vi "List_Inst_Positions.vi"() -> (0 "Position Info":string[][](array[string]))   [LabVIEW 2011]
uses:
  Anemometry/Anemometry Sub Vis/Globals/Meas_global.vi
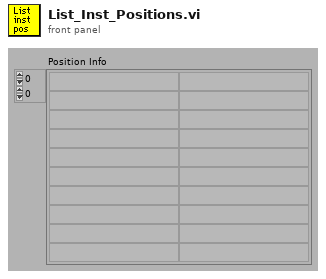
[diagram p1: front panel]
types:
  T1 = typedef "Analysis_info_cluster.ctl" = cluster{"Colour":u32, "Inst type":T2, "Inst name":string, "Symbol":string, "Code name":string, "Extra Info":string, "Inst Array":T3, "Index":i32, "Voltage Index":i32, "Extra Titles":string[], "Extra Values":string[], "Eng Values":dbl[], "Time (ms)":dbl[], "Voltage":dbl[], "U":dbl, "u^2":dbl, "u^3":dbl, "u^4":dbl, "Skew_u":dbl, "Kurt_u":dbl, "Sd Error in Mean":dbl, "% u'/U":dbl, "X":dbl, "Y":dbl, "Z":dbl, "Spectra":T4, "Autocorrelation":T4, "Timescale integral to 25%":dbl, "Sd Error in Variance":dbl, "Calib File":path, "Calib Constants":dbl[], "Histogram":T4, "Output Position":bool, "Full Stats":bool, "Weighting":dbl[]}
  T2 = typedef "Inst_type.ctl" = enum16{"Propeller anemometer", "Raw voltage", "Pressure Transducer", "Pitot-static tube", "Preston tube", "Hot wire", "Cross wire 1", "Cross wire 2", "Generic Linear", "Generic Polynomial", "Generic BackPoly", "Fast FID", "Thermocouple", "Cold wire", "Pulsed Wire", "LDA Vel", "LDA Tran time", "LDA Arr time"}
  T3 = typedef "Instrument_Array.ctl" = enum16{"PWA", "LDA", "Analogue"}
  T4 = typedef "XY_Plot_Cluster.ctl" = cluster{"First Name":string, "Second Name":string, "X axis name":string, "Y axis name":string, "X array":dbl[], "Y array":dbl[]}
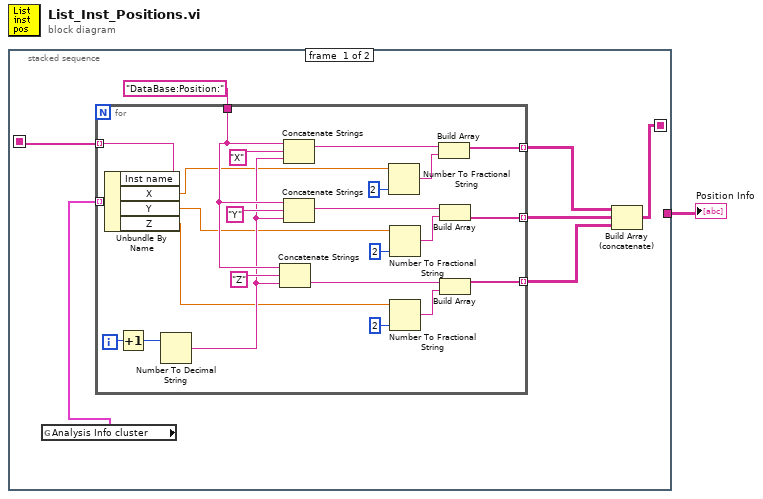
[diagram p0: block diagram]
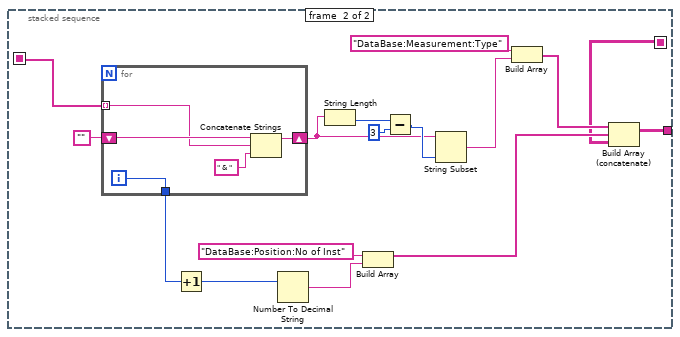
[diagram p2: hidden frame]
diagram:
  n1 = stacked-sequence {
    seq-local: [w4 _] -> [_ w34]
    seq-local: [w3 _] -> [_ w44]
    tunnel: [_ w33] -> w1
    frame #0 {
      n2 = global read "Meas_global.vi" "Analysis Info cluster"() -> (w2:T1[])
      n3 = for {
        tunnel: w2 -> [w32] mode=indexing
        tunnel: "DataBase:Position:" -> [w29]
        tunnel: [w13] -> w7 mode=indexing
        tunnel: [w12] -> w6 mode=indexing
        tunnel: [w11] -> w5 mode=indexing
        tunnel: [w9] -> w3 mode=indexing
        i -> [w30]
        n4 = Unbundle By Name(w32) -> ("Inst name"=w9:string, "X"=w22:dbl, "Y"=w16:dbl, "Z"=w15:dbl)
        n5 = Increment(x=w30) -> (x+1=w10:i32)
        n6 = Number To Decimal String(number=w10) -> (decimal integer string=w26:string)  [unwired: 1 out]
        n7 = Concatenate Strings(w29, "Z", w26) -> (w14:string)
        n8 = Concatenate Strings(w29, "X", w26) -> (w25:string)
        n9 = Concatenate Strings(w29, "Y", w26) -> (w17:string)
        n10 = Number To Fractional String(number=w22, precision (6)=i16 2) -> (F-format string=w23:string)  [unwired: 2 out]
        n11 = Number To Fractional String(number=w16, precision (6)=i16 2) -> (F-format string=w21:string)  [unwired: 2 out]
        n12 = Number To Fractional String(number=w15, precision (6)=i16 2) -> (F-format string=w18:string)  [unwired: 2 out]
        n13 = Build Array(w25, w23) -> (w12:string[])
        n14 = Build Array(w17, w21) -> (w13:string[])
        n15 = Build Array(w14, w18) -> (w11:string[])
      }
      n16 = Build Array (concatenate)(w6, w7, w5) -> (w4:string[][])
    }
    frame #1 {
      n17 = for {
        shift-right: [w52] -> w40
        shift-left: "" -> [w53]
        tunnel: w44 -> [w51] mode=indexing
        tunnel: [w49] -> w38
        i -> [w49]
        n18 = Concatenate Strings(w53, w51, " & ") -> (w52:string)
      }
      n19 = Increment(x=w38) -> (x+1=w37:i32)
      n20 = Number To Decimal String(number=w37) -> (decimal integer string=w47:string)  [unwired: 1 out]
      n21 = String Length(string=w40) -> (length=w43:i32)
      n22 = Build Array("DataBase:Position:No of Inst", w47) -> (w35:string[])
      n23 = Subtract(x=w43, y=3) -> (x-y=w41:i32)
      n24 = String Subset(string=w40, length (rest)=w41) -> (substring=w39:string)  [unwired: 1 out]
      n25 = Build Array("DataBase:Measurement:Type", w39) -> (w36:string[])
      n26 = Build Array (concatenate)(w36, w35, w34) -> (w33:string[][])
    }
  }
  "Position Info" <- w1
